vi "Realsense Cam Capture Start.vi"(8 "error in (no error)":errorcluster, 11 "Realsense Cam in":refnum<class "Realsense Cam.lvclass">) -> (0 "error out":errorcluster, 2 "Config Error":string, 3 "Realsense Cam out":refnum<class "Realsense Cam.lvclass">)   [LabVIEW 2018, in "Realsense Cam.lvclass"]
uses:
  Realsense Cam.lvclass
  Realsense Cam.lvclass/Realsense Cam.ctl
  Temp/realsense_labview_sdk/RealSense SDK2.11.0 for LabVIEW/libRealSense3.lvlib
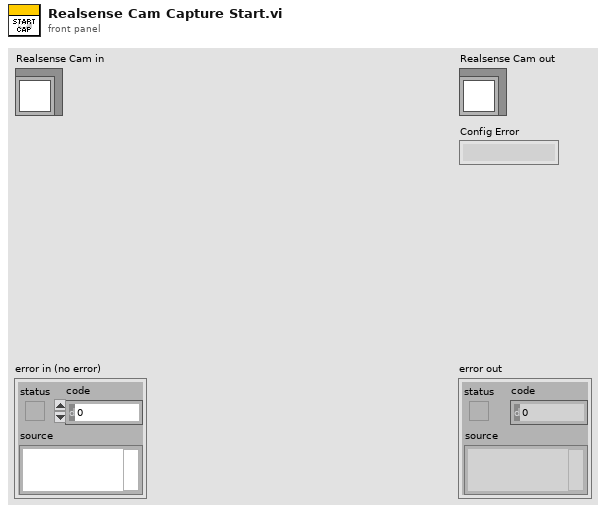
[diagram p1: front panel]
types:
  T1 = typedef "Realsense Cam.lvclass/Activated Stream STYP.ctl" = cluster{"Stream Type":T2, "Resolution":u16, "Profile Handle":u64, "Stream":T3}
  T2 = typedef "Realsense Cam.lvclass/Stream Types Enum STYP.ctl" = enum16{"Depth", "Left IR", "Right IR", "Color", "RGB Ext.", "Left IR Unrectified", "Right IR Unrectified"}
  T3 = typedef "Realsense Cam.lvclass/Stream STYP.ctl" = cluster{"Strings":string[], "Intrinsics":cluster{"width":i32, "height":i32, "fps":i32, "Profile":u64, "ppx":sgl, "ppy":sgl, "fx":sgl, "fy":sgl, "model":u32}[], "Current Data":cluster{"Depths":sgl[][], "Bytes":u8[], "Height":i32, "Width":i32}}
  T4 = cluster{"decimation filter queue":u64, "spatial filter queue":u64, "temporal filter queue":u64, "disparity_transforg_2_queue":u64, "disparity_transforg_1_queue":u64}
  T5 = cluster{"decimation filter block":u64, "spatial filter block":u64, "temporal filter block":u64, "disparity_transforg_2_block":u64, "disparity_transforg_1_block":u64}
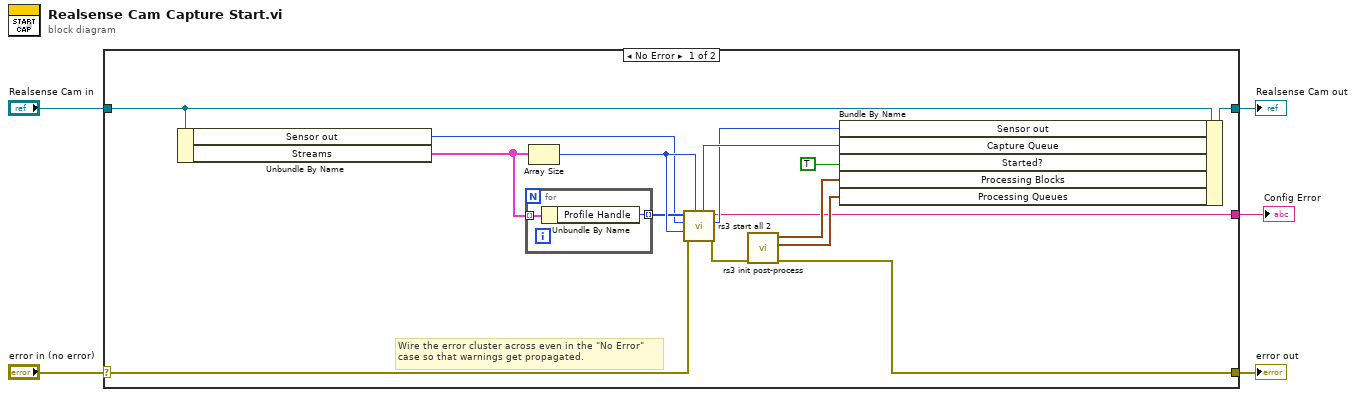
[diagram p0: block diagram]
diagram:
  n1 = case shown="No Error" "error in (no error)" {
    selector: "error in (no error)" -> [w11 w24]
    tunnel: [w10 w24] -> w4
    tunnel: [w6 w23] -> w2
    tunnel: "Realsense Cam in" -> [w16 w23]
    tunnel: [w7 _] -> w1
    frame No Error {
      # "Wire the error cluster across even in the \"No Error\"\ncase so that warnings get propagated."
      n2 = Unbundle By Name(w16) -> ("Sensor out"=w17:u64, "Streams"=w20:T1[])
      n3 = for {
        tunnel: w20 -> [w22] mode=indexing
        tunnel: [w21] -> w18 mode=indexing
        n4 = Unbundle By Name(w22) -> ("Profile Handle"=w21:u64)
      }
      n5 = Array Size(array=w20) -> (size(s)=w19:i32)
      n6 = call "rs3 start all 2.vi"("capacity"=w19, "error in (no error)"=w11, "Count of Streams"=w19, "Sensor in"=w17, "Stream profile array"=w18) -> ("error out"=w12:errorcluster, "sensor out"=w13:u64, "Config Error"=w7:string, "queue out"=w14:u64)  [unwired: 3 in]
      n7 = call "rs3 init post-process.vi"("error in (no error)"=w12) -> ("error out"=w10:errorcluster, "Processing Queues"=w8:T4, "Processing Blocks"=w9:T5)  [unwired: 8 in]
      n8 = Bundle By Name(cluster=w16, "Sensor out"=w13, "Capture Queue"=w14, "Started?"=TRUE ("Stream Data.Started?"), "Processing Blocks"=w9, "Processing Queues"=w8) -> (w6:refnum<class "Realsense Cam.lvclass">)
    }
    frame Error {
    }
  }
  "error out" <- w4
  "Realsense Cam out" <- w2
  "Config Error" <- w1
